vi "cw_5_3.vi"() -> ()   [LabVIEW 2022 SP3]
panel:
  in  "Array":bool[][](array[boolean])
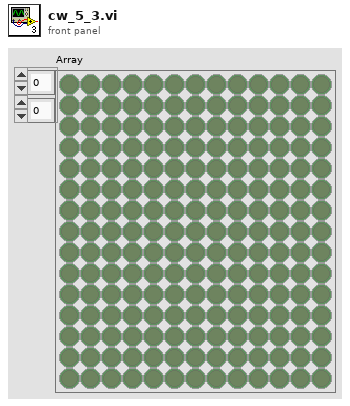
[diagram p1: front panel]
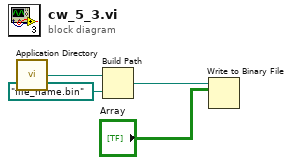
[diagram p0: block diagram]
diagram:
  n1 = call <vilib>:"Application Directory.vi"() -> ("Application Directory"=w4:path)
  n2 = Build Path(base path=w4, name or relative path=path "file_name.bin") -> (appended path=w2:path)
  n3 = Write to Binary File(file (use dialog)=w2, data="Array") -> ()  [unwired: 4 in, 3 out]
